vi "Set-motor-status.vi"(8 "error in (no error)":errorcluster, 10 "Status array":string[](array[string]), 11 "Object ref in":T1) -> (0 "error out":errorcluster, 3 "Object ref out":T1)   [LabVIEW 2013, in "PowderDeposition.lvlib" / "PD-Main.lvclass"]
uses:
  PD-Main.lvclass
  Object-reference.ctl
  PD-Main.lvclass/PD-Main.ctl
  Read Motors-status.vi
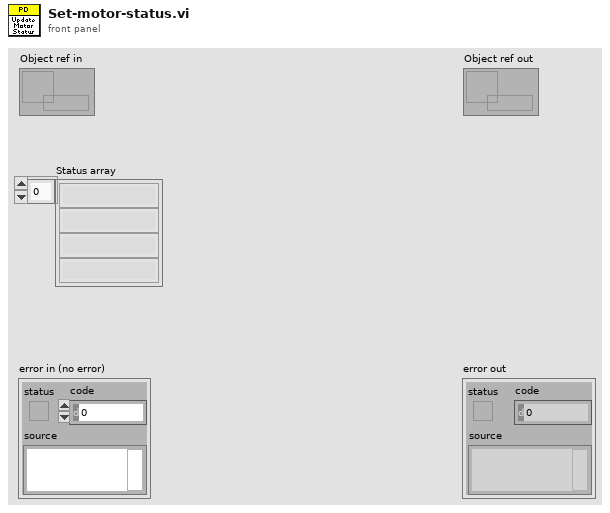
[diagram p1: front panel]
types:
  T1 = typedef "PowderDeposition.lvlib/PD-Main.lvclass/Object-reference.ctl" = refnum<data-value>
  T2 = cluster{"Status array[0]":string, "Status array[1]":string, "Status array[2]":string, "Status array[3]":string}
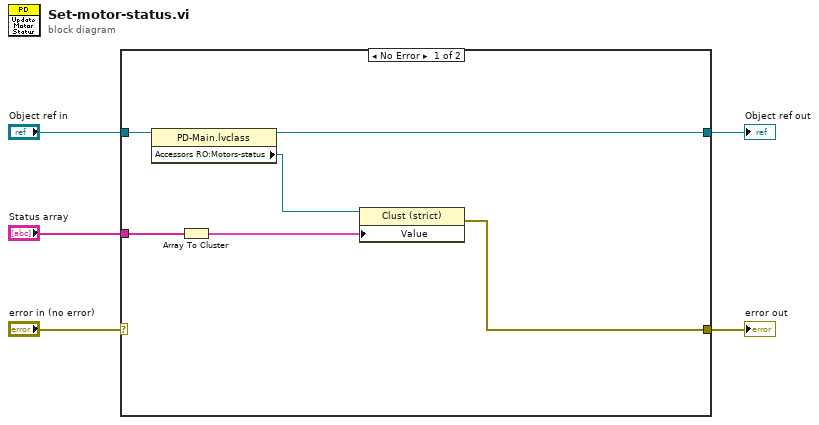
[diagram p0: block diagram]
diagram:
  n1 = case shown="No Error" "error in (no error)" {
    selector: "error in (no error)" -> [_ w13]
    tunnel: [w9 w13] -> w4
    tunnel: [w10 w12] -> w2
    tunnel: "Object ref in" -> [w11 w12]
    tunnel: "Status array" -> [w8 _]
    frame No Error {
      n2 = property class="PD-Main.lvclass"(reference=w11) -> (reference out=w10:T1, "Accessors RO:Motors-status"=w7:refnum<vi>)  [unwired: 1 in, 1 out]
      n3 = Array To Cluster(array=w8) -> (cluster=w6:T2)
      n4 = property class="Clust (strict)"(reference=w7, "Value"=w6) -> (error out=w9:errorcluster)  [unwired: 1 in, 1 out]
    }
    frame Error {
    }
  }
  "error out" <- w4
  "Object ref out" <- w2
